vi "json_labview_2012.vi"(8 "error in":errorcluster, 11 "Path":path) -> (0 "error out":errorcluster, 3 "data from JSON file":T1)   [LabVIEW 2016]
panel:
  out "Expected format":string
  out "JSON file content":string
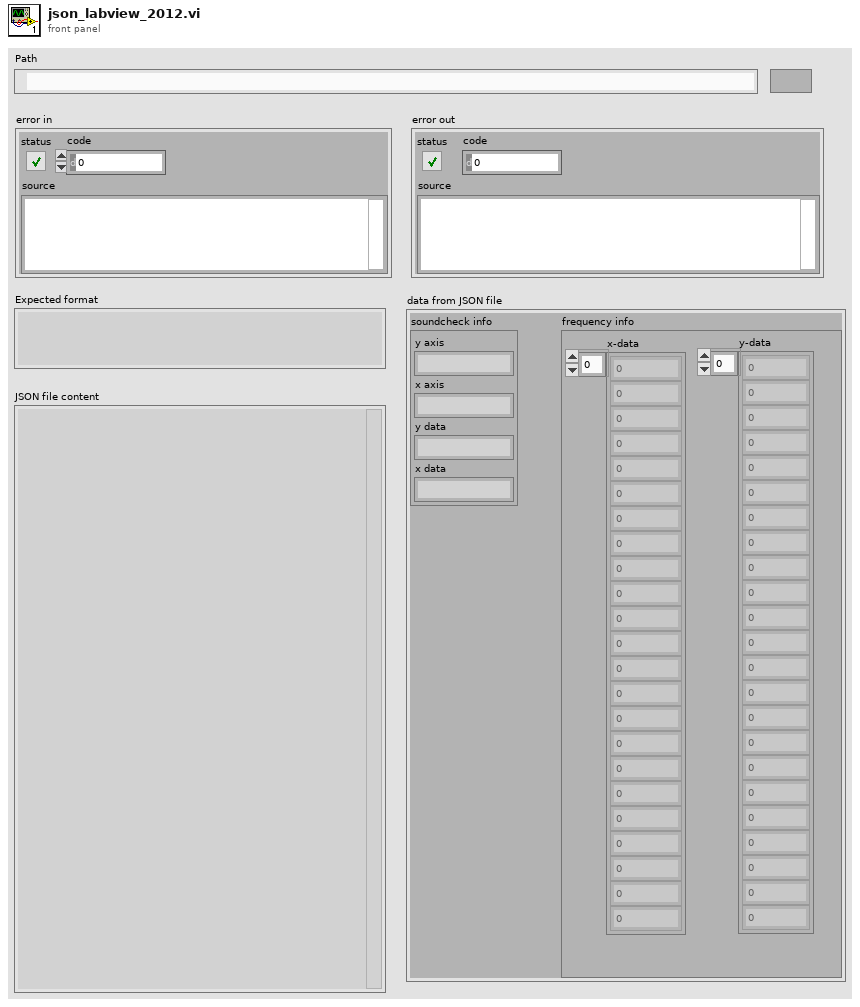
[diagram p1: front panel]
types:
  T1 = cluster{"frequency info":cluster{"y-data":dbl[], "x-data":dbl[]}, "soundcheck info":cluster{"y axis":string, "x axis":string, "y data":string, "x data":string}}
  T2 = enum16{"open", "replace", "create", "open or create", "replace or create", "replace or create with confirmation"}
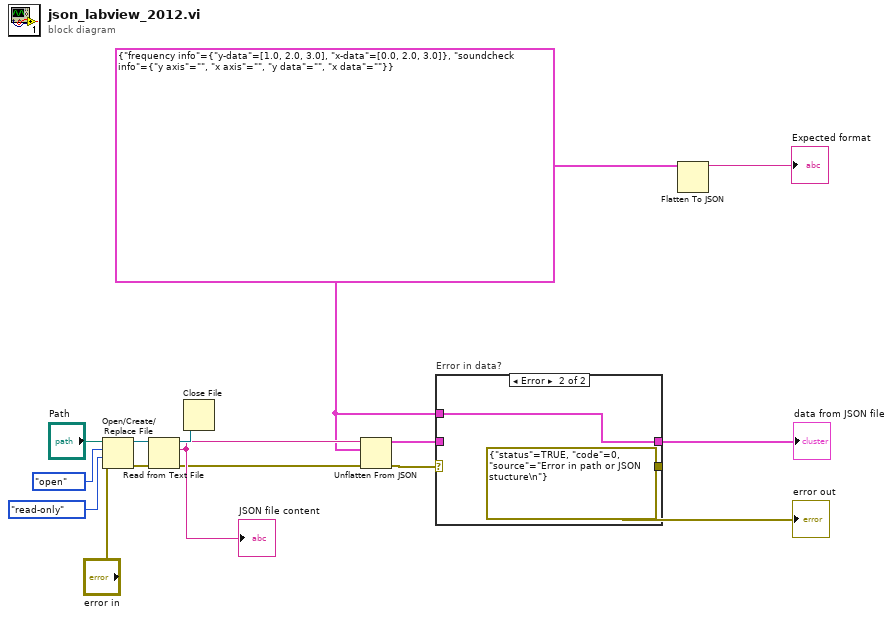
[diagram p0: block diagram]
diagram:
  w3 = T1 {"frequency info"={"y-data"=[1.0, 2.0, 3.0], "x-data"=[0.0, 2.0, 3.0]}, "soundcheck info"={"y axis"="", "x axis"="", "y data"="", "x data"=""}}
  n1 = Open/Create/Replace File(file path (use dialog)="Path", error in="error in", operation (0:open)=T2."open", access (0:read/write)=enum16{"read/write", "read-only", "write-only"}."read-only") -> (refnum out=w12:refnum<file>, error out=w11:errorcluster)  [unwired: 2 in, 1 out]
  n2 = Read from Text File(file (use dialog)=w12, error in=w11) -> (refnum out=w10:refnum<file>, text=w8:string, error out=w7:errorcluster)  [unwired: 2 in, 1 out]
  "JSON file content" <- w8
  n3 = Close File(refnum=w10) -> ()  [unwired: 1 in, 2 out]
  n4 = Unflatten From JSON(JSON string=w8, type and defaults=w3, error in (no error)=w7) -> (value=w4:T1, error out=w6:errorcluster)  [unwired: 4 in]
  n5 = case "Error in data?" shown="Error" w6 {
    selector: w6 -> [w16 _]
    tunnel: [w17 w19] -> w5
    tunnel: w4 -> [w17 _]
    tunnel: w3 -> [_ w19]
    tunnel: [w16 errorcluster {"status"=TRUE, "code"=0, "source"="Error in path or JSON stucture\n"} ("error out")] -> w1
    frame No Error {
    }
    frame Error {
    }
  }
  "data from JSON file" <- w5
  "error out" <- w1
  n6 = Flatten To JSON(anything=w3) -> (JSON string=→"Expected format":string)  [unwired: 2 in, 1 out]
